vi "RouthTest.vi"() -> ()   [LabVIEW 2019]
uses:
  <vilib>/imath/engines/lvmath2/RunTimeEngine/BuiltInFunctions/size/NIMS_I32Row=size(GRow).vi
  <instcachedir>/0/NIMS_I32Row=size(GRow)_E5C05C6B13124B29B774CC4F993D3C59.lvgen/NIMS_I32Row=size(GRow)_E5C05C6B13124B29B774CC4F993D3C59_000.vi
  <vilib>/imath/engines/lvmath2/RunTimeEngine/IndexRead/NIMS V(S).vi
  <instcachedir>/0/NIMS V(S)_0488751826AF41519A22953C041130DC.lvgen/NIMS V(S)_0488751826AF41519A22953C041130DC_002.vi
  <vilib>/imathl/engines/lvmath/Functions/Error Handling/Create Error.vi
  <vilib>/imath/engines/lvmath2/RunTimeEngine/BuiltInFunctions/zeros/NIMS_M=zeros(I32,I32).vi
  <vilib>/imath/engines/lvmath2/RunTimeEngine/RangeToken/NIMS_Range_R2 - Integer.vi
  <instcachedir>/0/NIMS_Range_R2 - Integer_5118B3908D7D4A9BA0DEB8EE73549D2D.lvgen/NIMS_Range_R2 - Integer_5118B3908D7D4A9BA0DEB8EE73549D2D_000.vi
  <vilib>/imath/engines/lvmath2/RunTimeEngine/CommandStatement/MC_CommandStatement_break.vi
  <vilib>/imath/engines/lvmath2/RunTimeSupport/NIMS_Error if Not Equal.vi
  <instcachedir>/0/NIMS_Error if Not Equal_559A38B1E9844760937E85B04C5ADA21.lvgen/NIMS_Error if Not Equal_559A38B1E9844760937E85B04C5ADA21_000.vi
  <vilib>/imath/engines/lvmath2/RunTimeEngine/BuiltInFunctions/rem/NIMS_rem_no checks.vi
  <instcachedir>/0/NIMS_rem_no checks_C77F7F87F9A543BB9CDCD173D9C96A12.lvgen/NIMS_rem_no checks_C77F7F87F9A543BB9CDCD173D9C96A12_008.vi
  <instcachedir>/0/NIMS V(S)_0488751826AF41519A22953C041130DC.lvgen/NIMS V(S)_0488751826AF41519A22953C041130DC_000.vi
  <vilib>/imath/engines/lvmath2/RunTimeEngine/IndexReplace/NIMS M(S,S)=S.vi
  <instcachedir>/0/NIMS M(S,S)=S_298DA19755FE42BBB9877D849ED339EF.lvgen/NIMS M(S,S)=S_298DA19755FE42BBB9877D849ED339EF_000.vi
  <vilib>/imath/engines/lvmath2/RunTimeEngine/ErrorHandling/NIMS_Create Error From Enums.vi
  <vilib>/imath/engines/lvmath2/RunTimeEngine/BuiltInFunctions/zeros/NIMS_V=zeros(I32,I32).vi
  <vilib>/imath/engines/lvmath2/RunTimeEngine/IndexReplace/NIMS V(S)=S.vi
  <instcachedir>/0/NIMS V(S)=S_B9932668475A4AEEB58CEEAB74E1195A.lvgen/NIMS V(S)=S_B9932668475A4AEEB58CEEAB74E1195A_000.vi
  <vilib>/imath/engines/lvmath2/RunTimeEngine/IndexRead/NIMS M(S,$).vi
  <instcachedir>/0/NIMS M(S,$)_F24F360562DE41D8BE234322A2E15C65.lvgen/NIMS M(S,$)_F24F360562DE41D8BE234322A2E15C65_000.vi
  <vilib>/imath/engines/lvmath2/RunTimeEngine/BuiltInFunctions/all/NIMS_all(GRowV).vi
  <vilib>/imath/engines/lvmath2/RunTimeEngine/IndexRead/NIMS M(S,S).vi
  <instcachedir>/0/NIMS M(S,S)_AC51E74150A542F7991B9634C66F3096.lvgen/NIMS M(S,S)_AC51E74150A542F7991B9634C66F3096_000.vi
  <vilib>/imath/engines/lvmath2/RunTimeEngine/BuiltInFunctions/eps/NIMS_eps.vi
  <vilib>/imath/engines/lvmath2/RunTimeEngine/RangeToken/NIMS_Range.vi
  <instcachedir>/0/NIMS_Range_0856D726B6B24596B614846B21C682A9.lvgen/NIMS_Range_0856D726B6B24596B614846B21C682A9_000.vi
  <instcachedir>/0/NIMS_Error if Not Equal_559A38B1E9844760937E85B04C5ADA21.lvgen/NIMS_Error if Not Equal_559A38B1E9844760937E85B04C5ADA21_001.vi
  <vilib>/imath/engines/lvmath2/RunTimeEngine/IndexRead/NIMS M(S,V).vi
  <instcachedir>/0/NIMS M(S,V)_5C1965D37F59432CA0E9661793EAFE90.lvgen/NIMS M(S,V)_5C1965D37F59432CA0E9661793EAFE90_000.vi
  <instcachedir>/0/NIMS_Range_0856D726B6B24596B614846B21C682A9.lvgen/NIMS_Range_0856D726B6B24596B614846B21C682A9_001.vi
  <vilib>/imath/engines/lvmath2/RunTimeEngine/ArithmeticOperatorToken/NIMS_ArithmeticOperator_times.vi
  <instcachedir>/0/NIMS_ArithmeticOperator_times_BC2A7BF92F8245379E8C6B3F6BDCD4B7.lvgen/NIMS_ArithmeticOperator_times_BC2A7BF92F8245379E8C6B3F6BDCD4B7_008.vi
  <vilib>/imath/engines/lvmath2/RunTimeEngine/IndexReplace/NIMS M(S,V)=V.vi
  <instcachedir>/0/NIMS M(S,V)=V_E83199AE38934AB3B484252ED68DE15E.lvgen/NIMS M(S,V)=V_E83199AE38934AB3B484252ED68DE15E_000.vi
  <vilib>/imath/engines/lvmath2/RunTimeEngine/RangeToken/NIMS_Range_R2 - Float.vi
  <instcachedir>/0/NIMS_Range_R2 - Float_34C0770B58484855BEFB6CBFA9AC9324.lvgen/NIMS_Range_R2 - Float_34C0770B58484855BEFB6CBFA9AC9324_000.vi
  <vilib>/imath/engines/lvmath2/RunTimeEngine/BuiltInFunctions/det/NIMS_det.vi
  <instcachedir>/0/NIMS_det_FC43403F6A814B2FA6A2876A6DC65E99.lvgen/NIMS_det_FC43403F6A814B2FA6A2876A6DC65E99_000.vi
  <vilib>/imath/engines/lvmath2/RunTimeEngine/NodeEndStatement/NIMS_NodeEndStatement_Output.vi
  <instcachedir>/0/NIMS_NodeEndStatement_Output_53EC0D466D134D7ABD903AC30B43404B.lvgen/NIMS_NodeEndStatement_Output_53EC0D466D134D7ABD903AC30B43404B_002.vi
  <vilib>/imath/engines/lvmath2/RunTimeEngine/ErrorHandling/NIMS_Finalize Error.vi
panel:
  out "resulting string":string
  out "Conclusion":string
  out "Number of roots\n in RHS plane":i16
  out "0, 1":i16[](array[numeric])
  out "Array 2":bool[](array[boolean])
  out "sign":dbl[](array[numeric])
  out "Array":dbl[](array[numeric])
  in  "poli":dbl[](array[numeric])
  out "Routh-Array":dbl[][](array[numeric])
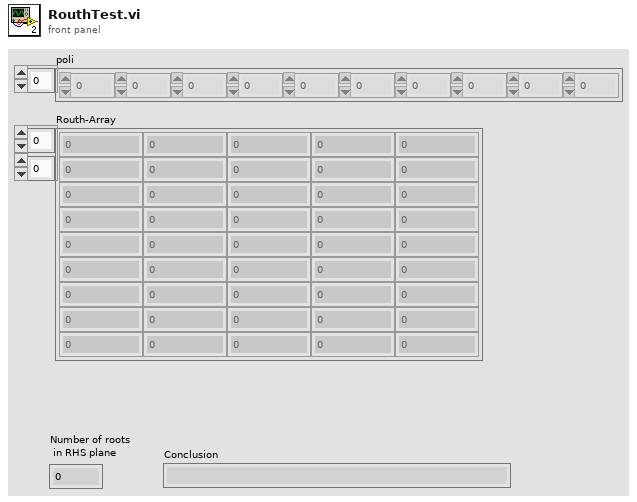
[diagram p1: front panel]
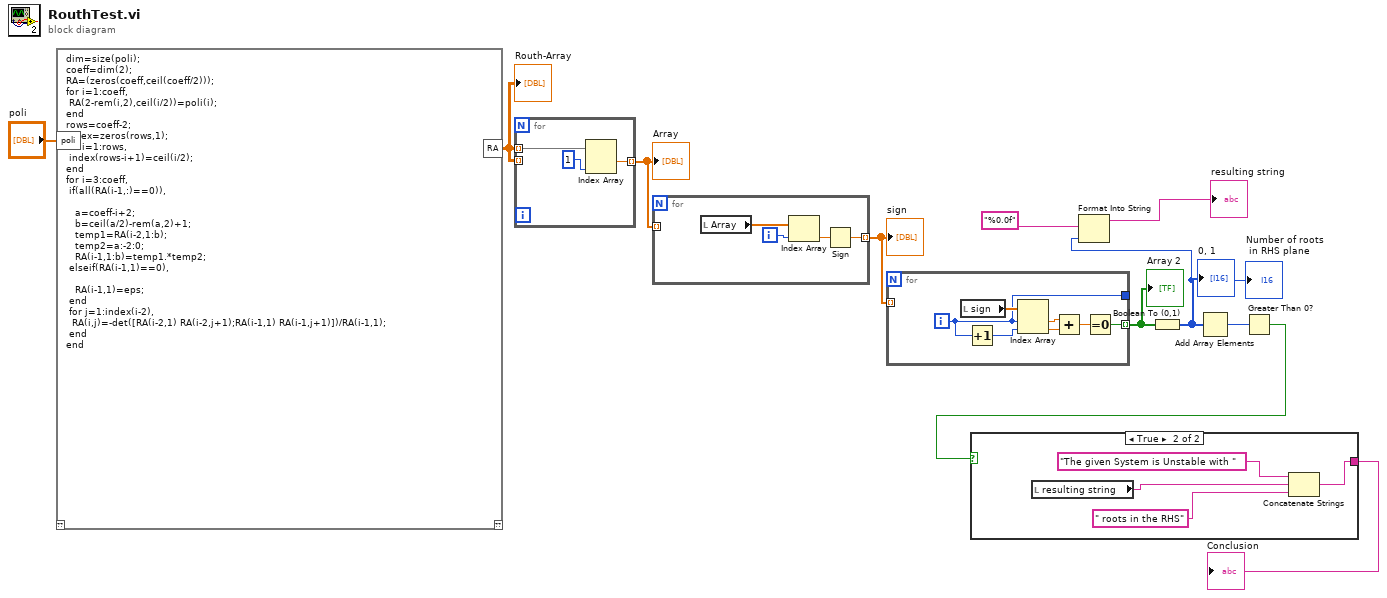
[diagram p0: block diagram]
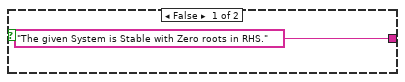
[diagram p2: hidden frame]
diagram:
  n1 = mathscript code="dim=size(poli);\t\t\t\ncoeff=dim(2);\t\t\t\t\nRA=(zeros(coeff,ceil(coeff/2)));\t \nfor i=1:coeff,\n\tRA(2-rem(i,2),ceil(i/2))=poli(i); \nend\nrows=coeff-2;\t\t\nindex=zeros(rows,1);\t\nfor i=1:rows,\n\tindex(rows-i+1)=ceil(i/2); \nend\nfor i=3:coeff,\t\t\t\n\tif(all(RA(i-1,:)==0)),\t\n\t\t\n\t\t\ta=coeff-i+2;\t\t\n\t\t\tb=ceil(a/2)-rem(a,2)+1; \n\t\t\ttemp1=RA(i-2,1:b);\t\n\t\t\ttemp2=a:-2:0;\t\n\t\t\tRA(i-1,1:b)=temp1.*temp2;\t\n\telseif(RA(i-1,1)==0),\t\t\n\t\t\n\t\t\tRA(i-1,1)=eps;\t\n\tend\n\tfor j=1:index(i-2),\t\n\t\tRA(i,j)=-det([RA(i-2,1) RA(i-2,j+1);RA(i-1,1) RA(i-1,j+1)])/RA(i-1,1);\n\tend\nend"("poli"="poli") -> ("RA"=w10:dbl[][])  [unwired: 1 in, 1 out]
  "Routh-Array" <- w10
  n2 = for {
    tunnel: w10 -> [w14] mode=indexing
    tunnel: w10 -> [_] mode=indexing
    tunnel: [w13] -> w9 mode=indexing
    n3 = Index Array(array=w14, index #2=1 ("index")) -> (element #1=w13:dbl)  [unwired: 1 in, 1 out]
  }
  "Array" <- w9
  n4 = for {
    tunnel: w9 -> [_] mode=indexing
    tunnel: [w15] -> w8 mode=indexing
    i -> [w18]
    n5 = local read "Array"() -> (w17:dbl[])
    n6 = Index Array(array=w17, index=w18) -> (element=w16:dbl)
    n7 = Sign(1:w16) -> (0:w15:dbl)
  }
  "sign" <- w8
  n8 = for {
    tunnel: w8 -> [_] mode=indexing
    tunnel: [w20] -> w7 mode=indexing
    tunnel: [w19] -> _
    i -> [w19]
    n9 = local read "sign"() -> (w25:dbl[])
    n10 = Increment(x=w19) -> (x+1=w24:i32)
    n11 = Index Array(array=w25, index #1=w19, index #2=w24) -> (element #1=w22:dbl, element #2=w23:dbl)
    n12 = Add(x=w22, y=w23) -> (x+y=w21:dbl)
    n13 = Equal To 0?(x=w21) -> (x = 0?=w20:bool)
  }
  "Array 2" <- w7
  n14 = Boolean To (0,1)(Boolean=w7) -> (0, 1=w6:i16[])
  "0, 1" <- w6
  n15 = Add Array Elements(numeric array=w6) -> (sum=w3:i16)
  "Number of roots\n in RHS plane" <- w3
  n16 = Format Into String(format string="%0.0f", w3) -> (resulting string=→"resulting string":string)  [unwired: 2 in, 1 out]
  n17 = Greater Than 0?(x=w3) -> (x > 0?=w1:bool)
  n18 = case shown="True" w1 {
    tunnel: ["The given System is Stable with Zero roots in RHS." ("String") w27] -> w5
    frame False {
    }
    frame True {
      n19 = local read "resulting string"() -> (w29:string)
      n20 = Concatenate Strings("The given System is Unstable with " ("String 2"), w29, " roots in the RHS") -> (w27:string)
    }
  }
  "Conclusion" <- w5
